vi "CRYDataView Main.vi"() -> ()   [LabVIEW 2013]
uses:
  <vilib>/Utility/miscctls.llb/LVRectTypeDef.ctl
  CRYView Global.vi
  CRYMainGlobal.vi
  CRYNew View Global.vi
  SubVI/CRYMain Sub Window Global.vi
panel:
  in  "pGraphMain VI Ref":refnum<vi>
  in  "Align":bool
  in  "bChangeState":bool
  in  "nIDFParent":i32
  in  "nSizeOver":i32
  in  "sAddGraphName":string="DataView"
  in  "Y2_Autoscale":bool
  in  "Y1_Autoscale":bool
  in  "X_Autoscale":bool
  in  "PreviewShowOnOff":bool
  in  "LegendShowOnOff":bool
  in  "Digital":bool
  in  "Intensity":bool
  in  "Octave":bool
  in  "Picture":bool
  in  "Polar":bool
  in  "Result":bool
  in  "Table":bool
  in  "Text":bool
  in  "Wave":bool
  in  "XY":bool
  in  "CursorShowOnOff":bool
  in  "sViewType":string="DataView"
  in  "sCloseMode":string="DataView"
  in  "AttachView":bool
  in  "sAddGraphLRAB":string="DataView"
  in  "Add Graph":bool
  in  "StateOut":bool
  in  "sTitle":string="DataView"
  in  "nIDV":i32
  in  "Revert":bool
  in  "Property":bool
  in  "TitleShowOnOff":bool
  in  "Save As":bool
  in  "Load":bool
  in  "stop":bool
  in  "cNewBootVIEW":T1
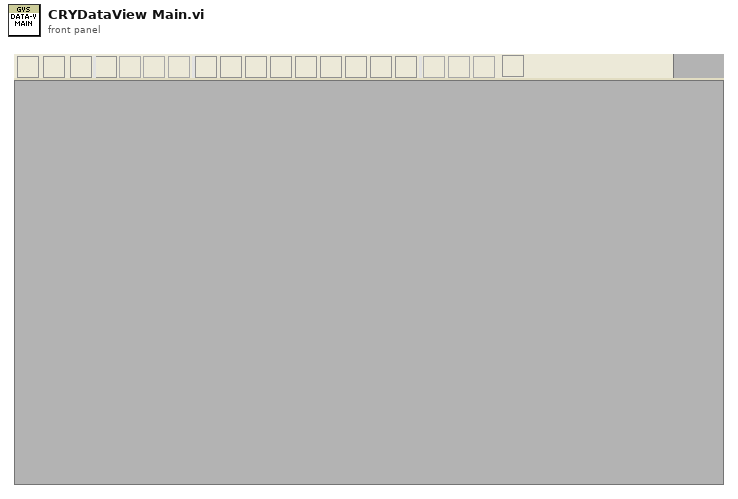
[diagram p1: front panel]
types:
  T1 = cluster{"sAction":string, "sType":string, "sQueueName":string, "sGraphName":string, "sData":string, "nData":i32, "pVIRef":refnum<vi>, "pSPRef":refnum<vi>}
  T2 = enum32{"English", "Chinese", "Korean", "Japanese", "Russian", "Chinese traditional"}
  T3 = typedef "LVRectTypeDef.ctl" = cluster{"Left":i16, "Top":i16, "Right":i16, "Bottom":i16}
  T4 = enum8{"Enabled", "Disabled", "Disabled and Grayed Out"}
  T5 = typedef "LVBoundsTypeDef.ctl" = cluster{"Width":u32, "Height":u32}
  T6 = cluster{"nID":i32, "sName":string, "sType":string, "sProperty":string, "sTemplet":string, "sDocking":string, "pVIRef":refnum<vi>, "pSPRef":refnum<vi>, "pRefTemplet":refnum<vi>, "pRefSplitter":refnum<vi>[], "nPosSplitter":i32[], "pRefSP":refnum<vi>[], "nSPID":i32[], "sSPDock":string[], "nIDFrame":i32[], "nIDPanel":i32[], "nActiveFrame":i32, "nCountFrame":i32, "cFrame":cluster{"nID":i32, "sName":string, "sType":string, "sTitle":string, "sIcon":string, "pVIRef":refnum<vi>, "pSPRef":refnum<vi>, "cWiin":cluster{"sName":string, "sType":string, "pVIRef":refnum<vi>, "sData":string}, "cTab":cluster{"sTitle":string, "sIcon":string, "pSpliter":refnum<vi>, "nAvtivePage":i32, "nIDPage":i32[], "nIDFrame":i32[]}, "sData":string}[], "sData":string, "sSplitterName":string[]}
  T7 = cluster{"nType":i32, "nParent":i32, "pVIW":refnum<vi>, "pSPW":refnum<vi>, "nTypeF":i32, "pVIF":refnum<vi>, "pSPF":refnum<vi>, "nIDSpliter":i32, "nProperty":i32, "Bound":T3, "nID":i32, "nData":i32, "sData":string, "pWVI":refnum<vi>, "sTitle":string, "cPages":cluster{"nPage":i32, "sTitle":string, "sIcon":string, "pVI":refnum<vi>, "nID":i32}[], "pTab":refnum<vi>, "nIDPages":i32[], "pSPT":refnum<vi>, "sTemp":string, "nDockID":i32, "nDockLR":i32, "sIcon":string}
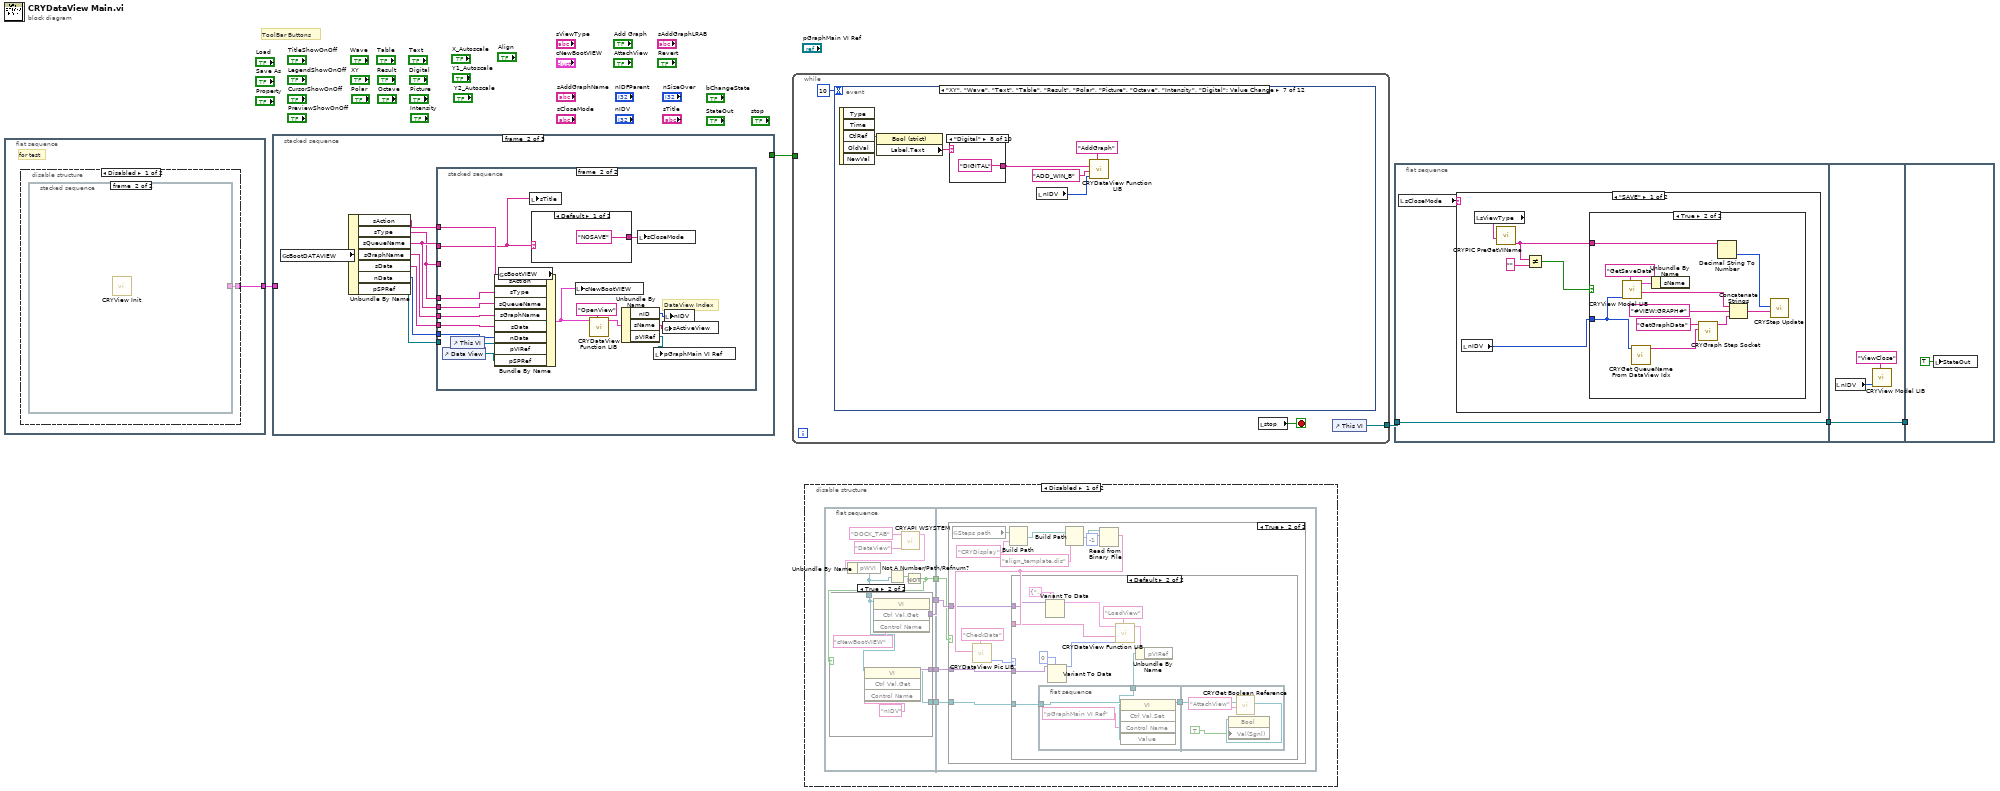
[diagram p0: block diagram]
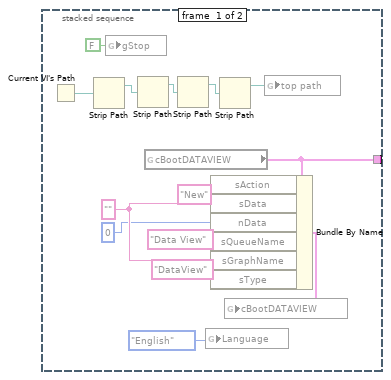
[diagram p6: hidden frame]
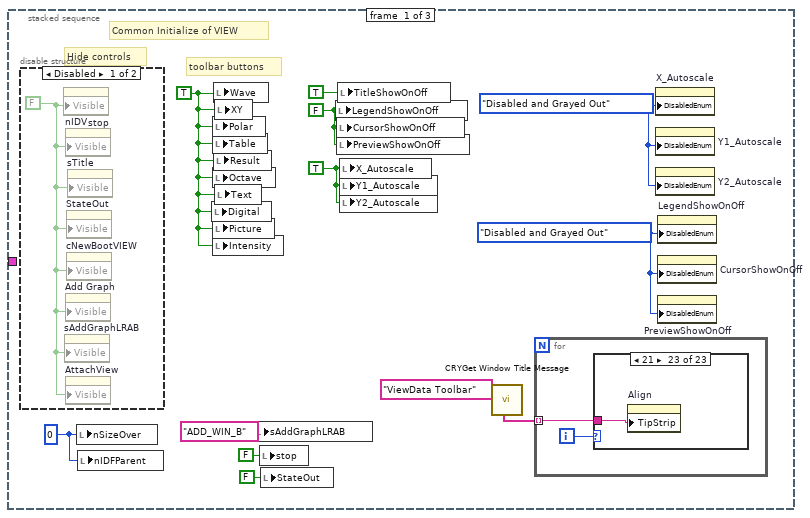
[diagram p10: hidden frame]
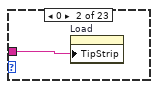
[diagram p13: hidden frame]
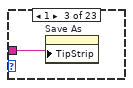
[diagram p14: hidden frame]
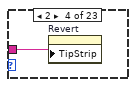
[diagram p15: hidden frame]
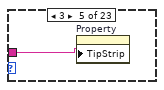
[diagram p16: hidden frame]
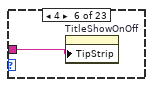
[diagram p17: hidden frame]
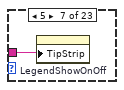
[diagram p18: hidden frame]
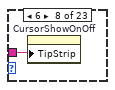
[diagram p19: hidden frame]
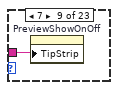
[diagram p20: hidden frame]
diagram:
  # "ToolBar Buttons"
  n1 = flat-sequence {
    tunnel: [w6] -> w1
    frame #0 {
      # "for test"
      n2 = disable-structure shown="Disabled" {
        disable-tunnel: [w7 _] -> w6
        frame Disabled {
          n3 = stacked-sequence {
            tunnel: [w8 _] -> w7
            frame #0 {
              w15 = "" ("sData")
              n4 = Current VI's Path() -> (path=w21:path)
              n5 = Strip Path(path=w21) -> (stripped path=w20:path)  [unwired: 1 out]
              n6 = global write "CRYMain Sub Window Global.vi" "gStop"(FALSE ("gStop")) -> ()
              n7 = Strip Path(path=w20) -> (stripped path=w19:path)  [unwired: 1 out]
              n8 = global read "CRYView Global.vi" "cBootDATAVIEW"() -> (w8:T1)
              n9 = Strip Path(path=w19) -> (stripped path=w18:path)  [unwired: 1 out]
              n10 = global write "CRYMainGlobal.vi" "Language"(T2."English" ("Language")) -> ()
              n11 = Bundle By Name(cluster=w8, "sAction"="New", "sData"=w15, "nData"=0, "sQueueName"="Data View", "sGraphName"=w15, "sType"="DataView") -> (w10:T1)
              n12 = Strip Path(path=w18) -> (stripped path=w17:path)  [unwired: 1 out]
              n13 = global write "CRYView Global.vi" "cBootDATAVIEW"(w10) -> ()
              n14 = global write "CRYMainGlobal.vi" "top path"(w17) -> ()
            }
            frame #1 {
              n15 = call "CRYView Init.vi"() -> ()  [unwired: 12 in]
            }
          }
        }
        frame Enabled {
        }
      }
    }
  }
  n16 = stacked-sequence {
    tunnel: [_ _ w97] -> w4
    tunnel: w1 -> [_ _ _]
    frame #0 {
      w23 = 0 ("nSizeOver")
      w24 = FALSE ("TitleShowOnOff")
      w25 = T4."Disabled and Grayed Out" ("Disabled")
      w26 = T4."Disabled and Grayed Out" ("Disabled")
      w27 = TRUE ("TitleShowOnOff")
      w29 = TRUE
      # "Hide controls"
      # "Common Initialize of VIEW"
      # "toolbar buttons"
      n17 = disable-structure shown="Disabled" {
        frame Disabled {
          w34 = FALSE
          n18 = property on="stop" class="Bool (strict)"("Visible"=w34) -> ()  [unwired: 2 in, 2 out]
          n19 = property on="sAddGraphLRAB" class="Str"("Visible"=w34) -> ()  [unwired: 2 in, 2 out]
          n20 = property on="nIDV" class="DigNum (strict)"("Visible"=w34) -> ()  [unwired: 2 in, 2 out]
          n21 = property on="Add Graph" class="Bool (strict)"("Visible"=w34) -> ()  [unwired: 2 in, 2 out]
          n22 = property on="AttachView" class="Bool (strict)"("Visible"=w34) -> ()  [unwired: 2 in, 2 out]
          n23 = property on="StateOut" class="Bool (strict)"("Visible"=w34) -> ()  [unwired: 2 in, 2 out]
          n24 = property on="cNewBootVIEW" class="Clust (strict)"("Visible"=w34) -> ()  [unwired: 2 in, 2 out]
          n25 = property on="sTitle" class="Str"("Visible"=w34) -> ()  [unwired: 2 in, 2 out]
        }
        frame Enabled {
        }
      }
      n26 = local write "nSizeOver"(w23) -> ()
      n27 = local write "nIDFParent"(w23) -> ()
      n28 = local write "Digital"(w29) -> ()
      n29 = local write "Polar"(w29) -> ()
      n30 = local write "Table"(w29) -> ()
      n31 = local write "Octave"(w29) -> ()
      n32 = local write "Picture"(w29) -> ()
      n33 = local write "Intensity"(w29) -> ()
      n34 = local write "Wave"(w29) -> ()
      n35 = local write "Result"(w29) -> ()
      n36 = local write "XY"(w29) -> ()
      n37 = local write "Text"(w29) -> ()
      n38 = local write "sAddGraphLRAB"("ADD_WIN_B" ("sAddGraphLRAB")) -> ()
      n39 = local write "stop"(FALSE ("stop")) -> ()
      n40 = local write "StateOut"(FALSE ("StateOut")) -> ()
      n41 = local write "LegendShowOnOff"(w24) -> ()
      n42 = local write "CursorShowOnOff"(w24) -> ()
      n43 = local write "PreviewShowOnOff"(w24) -> ()
      n44 = local write "TitleShowOnOff"(TRUE ("TitleShowOnOff")) -> ()
      n45 = local write "X_Autoscale"(w27) -> ()
      n46 = local write "Y1_Autoscale"(w27) -> ()
      n47 = local write "Y2_Autoscale"(w27) -> ()
      n48 = call "CRYGet Window Title Message.vi"("Kind"="ViewData Toolbar") -> ("Tip Strip"=w31:string[])  [unwired: 5 in, 5 out]
      n49 = for {
        tunnel: w31 -> [w35] mode=indexing
        i -> [w36]
        n50 = case shown="21" w36 {
          tunnel: w35 -> [_ w37 w38 w39 w40 w41 w42 w43 w44 w45 w46 w47 w48 w49 w50 w51 w52 w53 w54 w55 w56 w57 w58]
          frame Default {
          }
          frame 0 {
            n51 = property on="Load" class="Bool (strict)"("TipStrip"=w37) -> ()  [unwired: 2 in, 2 out]
          }
          frame 1 {
            n52 = property on="Save As" class="Bool (strict)"("TipStrip"=w38) -> ()  [unwired: 2 in, 2 out]
          }
          frame 2 {
            n53 = property on="Revert" class="Bool (strict)"("TipStrip"=w39) -> ()  [unwired: 2 in, 2 out]
          }
          frame 3 {
            n54 = property on="Property" class="Bool (strict)"("TipStrip"=w40) -> ()  [unwired: 2 in, 2 out]
          }
          frame 4 {
            n55 = property on="TitleShowOnOff" class="Bool (strict)"("TipStrip"=w41) -> ()  [unwired: 2 in, 2 out]
          }
          frame 5 {
            n56 = property on="LegendShowOnOff" class="Bool (strict)"("TipStrip"=w42) -> ()  [unwired: 2 in, 2 out]
          }
          frame 6 {
            n57 = property on="CursorShowOnOff" class="Bool (strict)"("TipStrip"=w43) -> ()  [unwired: 2 in, 2 out]
          }
          frame 7 {
            n58 = property on="PreviewShowOnOff" class="Bool (strict)"("TipStrip"=w44) -> ()  [unwired: 2 in, 2 out]
          }
          frame 8 {
            n59 = property on="Wave" class="Bool (strict)"("TipStrip"=w45) -> ()  [unwired: 2 in, 2 out]
          }
          frame 9 {
            n60 = property on="XY" class="Bool (strict)"("TipStrip"=w46) -> ()  [unwired: 2 in, 2 out]
          }
          frame 10 {
            n61 = property on="Polar" class="Bool (strict)"("TipStrip"=w47) -> ()  [unwired: 2 in, 2 out]
          }
          frame 11 {
            n62 = property on="Table" class="Bool (strict)"("TipStrip"=w48) -> ()  [unwired: 2 in, 2 out]
          }
          frame 12 {
            n63 = property on="Result" class="Bool (strict)"("TipStrip"=w49) -> ()  [unwired: 2 in, 2 out]
          }
          frame 13 {
            n64 = property on="Octave" class="Bool (strict)"("TipStrip"=w50) -> ()  [unwired: 2 in, 2 out]
          }
          frame 14 {
            n65 = property on="Text" class="Bool (strict)"("TipStrip"=w51) -> ()  [unwired: 2 in, 2 out]
          }
          frame 15 {
            n66 = property on="Digital" class="Bool (strict)"("TipStrip"=w52) -> ()  [unwired: 2 in, 2 out]
          }
          frame 16 {
            n67 = property on="Picture" class="Bool (strict)"("TipStrip"=w53) -> ()  [unwired: 2 in, 2 out]
          }
          frame 17 {
            n68 = property on="Intensity" class="Bool (strict)"("TipStrip"=w54) -> ()  [unwired: 2 in, 2 out]
          }
          frame 18 {
            n69 = property on="X_Autoscale" class="Bool (strict)"("TipStrip"=w55) -> ()  [unwired: 2 in, 2 out]
          }
          frame 19 {
            n70 = property on="Y1_Autoscale" class="Bool (strict)"("TipStrip"=w56) -> ()  [unwired: 2 in, 2 out]
          }
          frame 20 {
            n71 = property on="Y2_Autoscale" class="Bool (strict)"("TipStrip"=w57) -> ()  [unwired: 2 in, 2 out]
          }
          frame 21 {
            n72 = property on="Align" class="Bool (strict)"("TipStrip"=w58) -> ()  [unwired: 2 in, 2 out]
          }
        }
      }
      n73 = property on="X_Autoscale" class="Bool (strict)"("DisabledEnum"=w26) -> ()  [unwired: 2 in, 2 out]
      n74 = property on="Y1_Autoscale" class="Bool (strict)"("DisabledEnum"=w26) -> ()  [unwired: 2 in, 2 out]
      n75 = property on="Y2_Autoscale" class="Bool (strict)"("DisabledEnum"=w26) -> ()  [unwired: 2 in, 2 out]
      n76 = property on="LegendShowOnOff" class="Bool (strict)"("DisabledEnum"=w25) -> ()  [unwired: 2 in, 2 out]
      n77 = property on="CursorShowOnOff" class="Bool (strict)"("DisabledEnum"=w25) -> ()  [unwired: 2 in, 2 out]
      n78 = property on="PreviewShowOnOff" class="Bool (strict)"("DisabledEnum"=w25) -> ()  [unwired: 2 in, 2 out]
    }
    frame #1 {
      n79 = global read "CRYView Global.vi" "cBootDATAVIEW"() -> (w59:T1)
      n80 = Unbundle By Name(w59) -> ("sAction"=w62:string, "sType"=w61:string, "sQueueName"=w66:string, "sGraphName"=w65:string, "sData"=w64:string, "nData"=w63:i32, "pSPRef"=w60:refnum<vi>)
      n81 = stacked-sequence {
        tunnel: w62 -> [_ w86]
        tunnel: w66 -> [_ w79]
        tunnel: w63 -> [_ w90]
        tunnel: w64 -> [_ w91]
        tunnel: w65 -> [_ w92]
        tunnel: w66 -> [_ w93]
        tunnel: w61 -> [_ w94]
        tunnel: w61 -> [_ _]
        tunnel: w60 -> [w69 _]
        frame #0 {
          n82 = property class="SubPnl"(reference=w69) -> (error out=w68:errorcluster, "Bounds"=w67:T5)  [unwired: 1 in, 1 out]
          n83 = case shown="No Error" w68 {
            tunnel: w67 -> [w77 _]
            frame No Error {
              w72 = i16 0 ("Left")
              n84 = Unbundle By Name(w77) -> ("Width"=w74:u32, "Height"=w73:u32)
              n85 = Bundle By Name(cluster=T3 {"Left"=0, "Top"=0, "Right"=0, "Bottom"=0} ("Front Panel Window:Panel Bounds"), "Left"=w72, "Top"=w72, "Right"=w74, "Bottom"=w73) -> (w71:T3)
              n86 = control-ref of="This VI"() -> (w76:refnum<vi>)
              n87 = property class="VI"(reference=w76, "Front Panel.PanelBounds"=w71) -> (error out=w70:errorcluster)  [unwired: 1 in, 1 out]
              n88 = case shown="No Error" w70 {
                frame No Error {
                }
                frame Error {
                }
              }
            }
            frame Error {
            }
          }
        }
        frame #1 {
          # "DataView Index"
          n89 = control-ref of="Data View"() -> (w88:refnum<vi>)
          n90 = control-ref of="This VI"() -> (w84:refnum<vi>)
          n91 = global read "CRYView Global.vi" "cBootVIEW"() -> (w89:T1)
          n92 = Bundle By Name(cluster=w89, "sAction"=w86, "sType"=w94, "sQueueName"=w93, "sGraphName"=w92, "sData"=w91, "nData"=w90, "pVIRef"=w84, "pSPRef"=w88) -> (w87:T1)
          n93 = local write "sTitle"(w79) -> ()
          n94 = case shown="Default" w79 {
            tunnel: ["NOSAVE" "SAVE"] -> w85
            frame Default {
            }
            frame "ViewStep" {
            }
          }
          n95 = local write "cNewBootVIEW"(w87) -> ()
          n96 = call "CRYDataView Function LIB.vi"("sAction"="OpenView", "cBootVIEW"=w87) -> ("cView_Out"=w82:T6)  [unwired: 7 in, 2 out]
          n97 = Unbundle By Name(w82) -> ("nID"=w81:i32, "sName"=w80:string, "pVIRef"=w78:refnum<vi>)
          n98 = local write "sCloseMode"(w85) -> ()
          n99 = local write "pGraphMain VI Ref"(w78) -> ()
          n100 = global write "CRYView Global.vi" "sActiveView"(w80) -> ()
          n101 = local write "nIDV"(w81) -> ()
        }
      }
    }
    frame #2 {
      w97 = TRUE
      n102 = local write "StateOut"(w97) -> ()
    }
  }
  n103 = while {
    tunnel: [w99] -> w5
    tunnel: w4 -> [_]
    stop <- w98 stop-if-true
    n104 = event shown="[6] \"XY\", \"Wave\", \"Text\", \"Table\", \"Result\", \"Polar\", \"Picture\", \"Octave\", \"Intensity\", \"Digital\": Value Change" {
      selector: _ -> [_ _ _ _ _ _ _ _ _ _ _ _]
      dyn-events: _ -> [_ _ _ _ _ _ _ _ _ _ _ _]
      timeout: 10 -> [_ _ _ _ _ _ _ _ _ _ _ _]
      event Timeout {
        n105 = event-data() -> ()  [unwired: 1 in, 2 out]
      }
      event "Load": Value Change {
        n106 = event-data() -> ()  [unwired: 1 in, 5 out]
        n107 = global read "CRYMainGlobal.vi" "Steps path"() -> (w104:path)
        n108 = Build Path(base path=w104, name or relative path="CRYDisplay") -> (appended path=w103:path)
        n109 = call "CRYStep Read.vi"("Category Name"="Display" ("Step File Name"), "Step File Path"=w103) -> ("status"=w101:bool, "Flatten Step"=w102:string)  [unwired: 2 in, 4 out]
        n110 = case shown="True" w101 {
          tunnel: w102 -> [_ w107]
          frame False {
          }
          frame True {
            n111 = call "CRYDataView Pic LIB.vi"("sAction"="CheckData", "sOption"=w107) -> ("nData_Out"=w108:i32)  [unwired: 7 in, 2 out]
            n112 = case shown="Default" w108 {
              tunnel: w107 -> [_ w114]
              frame -1 {
              }
              frame Default {
                n113 = local read "nIDV"() -> (w112:i32)
                n114 = local read "cNewBootVIEW"() -> (w113:T1)
                n115 = call "CRYDataView Function LIB.vi"("sAction"="LoadView", "nData"=w112, "sData"=w114, "cBootVIEW"=w113) -> ("cView_Out"=w111:T6)  [unwired: 5 in, 2 out]
                n116 = Unbundle By Name(w111) -> ("pVIRef"=w110:refnum<vi>)
                n117 = flat-sequence {
                  tunnel: w110 -> [w116]
                  frame #0 {
                    n118 = local write "pGraphMain VI Ref"(w116) -> ()
                  }
                  frame #1 {
                    n119 = property on="AttachView" class="Bool (strict)"("Val(Sgnl)"=TRUE ("Value (Signaling)")) -> ()  [unwired: 2 in, 2 out]
                  }
                }
              }
            }
          }
        }
      }
      event "Save As": Value Change {
        n120 = event-data() -> ()  [unwired: 1 in, 5 out]
        n121 = local read "sViewType"() -> (w118:string)
        n122 = local read "nIDV"() -> (w119:i32)
        n123 = call "CRYDataView Function LIB.vi"("sAction"="SaveView", "nData"=w119, "sOption"=w118) -> ()  [unwired: 6 in, 3 out]
      }
      event "Revert": Value Change {
        n124 = event-data() -> ()  [unwired: 1 in, 5 out]
        n125 = local read "cNewBootVIEW"() -> (w121:T1)
        n126 = local read "nIDV"() -> (w122:i32)
        n127 = call "CRYDataView Function LIB.vi"("sAction"="ReloadView", "nData"=w122, "cBootVIEW"=w121) -> ()  [unwired: 6 in, 3 out]
      }
      event "TitleShowOnOff": Value Change {
        n128 = event-data() -> ()  [unwired: 1 in, 5 out]
        n129 = local read "nIDV"() -> (w124:i32)
        n130 = call "CRYDataView Function LIB.vi"("sAction"="TitleBarOnOff", "nData"=w124) -> ()  [unwired: 7 in, 3 out]
      }
      event "CursorShowOnOff", "LegendShowOnOff", "PreviewShowOnOff", "Property": Value Change {
        n131 = event-data() -> ("CtlRef"=w137:refnum<vi>, "OldVal"=w129:bool)  [unwired: 1 in, 3 out]
        n132 = property class="Bool (strict)"(reference=w137) -> ("Label.Text"=w136:string)  [unwired: 1 in, 2 out]
        n133 = local read "nIDV"() -> (w126:i32)
        n134 = case shown="\"CursorShowOnOff\"" w136 {
          tunnel: ["LEGEND_VIEW" ("input 1") "CURSOR_VIEW" ("input 1") "PREVIEW_VIEW" ("input 1") "DA_PROPERTY" ("input 1")] -> w132
          frame "LegendShowOnOff", Default {
          }
          frame "CursorShowOnOff" {
          }
          frame "PreviewShowOnOff" {
          }
          frame "Property" {
          }
        }
        n135 = Select(t=1, s=w129, f=-1) -> (s? t:f=w128:i32)
        n136 = call "CRYGet QueueName From DataView Idx.vi"("DataView Idx"=w126) -> ("DataView sQueueName"=w127:string)  [unwired: 10 in]
        n137 = Obtain Queue(name (unnamed)=w127, element data type="" ("Action Type")) -> (queue out=w133:refnum<queue>)  [unwired: 3 in, 2 out]
        n138 = Format Into String(w132, w132, w128, w126) -> (resulting string=w134:string)  [unwired: 3 in, 1 out]
        n139 = Enqueue Element(queue=w133, element=w134) -> ()  [unwired: 1 in, 4 out]
      }
      event "XY", "Wave", "Text", "Table", "Result", "Polar", "Picture", "Octave", "Intensity", "Digital": Value Change {
        n140 = event-data() -> ("CtlRef"=w142:refnum<vi>)  [unwired: 1 in, 4 out]
        n141 = property class="Bool (strict)"(reference=w142) -> ("Label.Text"=w143:string)  [unwired: 1 in, 2 out]
        n142 = case shown="\"Digital\"" w143 {
          tunnel: ["WAVE" "XY" "POLAR" "TABLE" "RESULT" "OCTAVE" "TEXT" "DIGITAL" "PICTURE" "INTENSITY"] -> w144
          frame "Wave", Default {
          }
          frame "XY" {
          }
          frame "Polar" {
          }
          frame "Table" {
          }
          frame "Result" {
          }
          frame "Octave" {
          }
          frame "Text" {
          }
          frame "Digital" {
          }
          frame "Picture" {
          }
          frame "Intensity" {
          }
        }
        n143 = local read "nIDV"() -> (w147:i32)
        n144 = call "CRYDataView Function LIB.vi"("sAction"="AddGraph", "nData"=w147, "sData"="ADD_WIN_B", "sOption"=w144) -> ()  [unwired: 5 in, 3 out]
      }
      event "X_Autoscale", "Y1_Autoscale", "Y2_Autoscale": Value Change {
        n145 = event-data() -> ("CtlRef"=w161:refnum<vi>)  [unwired: 1 in, 4 out]
        n146 = property class="Bool (strict)"(reference=w161) -> ("Label.Text"=w167:string)  [unwired: 1 in, 2 out]
        n147 = local read "nIDV"() -> (w159:i32)
        n148 = property class="Bool (strict)"(reference=w161) -> ("Value"=w162:bool)  [unwired: 1 in, 2 out]
        n149 = case shown="\"X_Autoscale\", Default" w167 {
          tunnel: ["X_AUTOSCALE" ("input 1") "Y1_AUTOSCALE" ("input 1") "Y2_AUTOSCALE" ("input 1")] -> w163
          frame "X_Autoscale", Default {
          }
          frame "Y1_Autoscale" {
          }
          frame "Y2_Autoscale" {
          }
        }
        n150 = Not(x=w162) -> (.not. x?=w160:bool)
        n151 = call "CRYGet QueueName From DataView Idx.vi"("DataView Idx"=w159) -> ("DataView sQueueName"=w158:string)  [unwired: 10 in]
        n152 = Select(t=1, s=w160, f=-1) -> (s? t:f=w164:i32)
        n153 = flat-sequence {
          tunnel: w163 -> [w171]
          tunnel: w158 -> [w170]
          tunnel: w164 -> [w169]
          tunnel: w159 -> [w168]
          frame #0 {
            n154 = Obtain Queue(name (unnamed)=w170, element data type="" ("Action Type")) -> (queue out=w172:refnum<queue>)  [unwired: 3 in, 2 out]
            n155 = Format Into String(w171, w171, w169, w168) -> (resulting string=w173:string)  [unwired: 3 in, 1 out]
            n156 = Enqueue Element(queue=w172, element=w173) -> ()  [unwired: 1 in, 4 out]
          }
        }
      }
      event "Align": Value Change {
        n157 = event-data() -> ()  [unwired: 1 in, 5 out]
        n158 = flat-sequence {
          frame #0 {
            n159 = global write "CRYNew View Global.vi" "g_WaitFlag"(TRUE ("g_WaitFlag")) -> ()
          }
          frame #1 {
            w180 = "VIEW_DATA_VIEW_TEMPLATE" ("input 1")
            w181 = 0 ("input 3")
            n160 = Obtain Queue(name (unnamed)="CRYMAIN_ACTION" ("YAxisTitle"), element data type="" ("Action Type")) -> (queue out=w179:refnum<queue>)  [unwired: 3 in, 2 out]
            n161 = Format Into String(w180, w180, w181, w181) -> (resulting string=w182:string)  [unwired: 3 in, 1 out]
            n162 = Enqueue Element(queue=w179, element=w182) -> ()  [unwired: 1 in, 4 out]
          }
        }
      }
      event "AttachView": Value Change {
        # "Fit problem"
        n163 = event-data() -> ()  [unwired: 1 in, 5 out]
        n164 = local read "pGraphMain VI Ref"() -> (w185:refnum<vi>)
        n165 = control-ref of="Data View"() -> (w186:refnum<vi>)
        n166 = invoke class="SubPnl" method="Insert VI"(reference=w186, "VI Ref"=w185) -> (reference out=w188:refnum<vi>, error out=w187:errorcluster)  [unwired: 2 in, 2 out]
        n167 = invoke class="SubPnl" method="FitControlToPane"(reference=w188, error in=w187) -> ()  [unwired: 1 in, 3 out]
      }
      event "bChangeState": Value Change {
        n168 = event-data() -> ("NewVal"=w193:bool)  [unwired: 1 in, 4 out]
        n169 = case shown="False" w193 {
          tunnel: [T4."Enabled" ("Disabled") T4."Disabled and Grayed Out" ("Disabled")] -> w192
          frame False {
          }
          frame True {
          }
        }
        n170 = control-ref of="Load"() -> (w191:refnum<vi>)
        n171 = control-ref of="Save As"() -> (w190:refnum<vi>)
        n172 = control-ref of="Property"() -> (w189:refnum<vi>)
        n173 = Build Array(w191, w190, w189) -> (w194:refnum<vi>[])
        n174 = for {
          tunnel: w194 -> [w196] mode=indexing
          tunnel: w192 -> [w195]
          n175 = property class="Bool (strict)"(reference=w196, "DisabledEnum"=w195) -> ()  [unwired: 1 in, 2 out]
        }
      }
      event Pane Size {
        w201 = 24
        n176 = event-data() -> ()  [unwired: 1 in, 5 out]
        n177 = local read "nSizeOver"() -> (w199:i32)
        n178 = control-ref of="Splitter"() -> (w200:refnum<vi>)
        n179 = property class="Splitter"(reference=w200) -> (reference out=w202:refnum<vi>, "Position"=w204:i32)  [unwired: 1 in, 1 out]
        n180 = Less?(x=w204, y=w201) -> (x < y?=w203:bool)
        n181 = case shown="True" w203 {
          tunnel: w202 -> [_ w249]
          tunnel: w201 -> [_ w251]
          tunnel: w199 -> [w205 _]
          frame False {
            n182 = disable-structure shown="Disabled" {
              disable-tunnel: w205 -> [w206 _]
              frame Disabled {
                n183 = case shown="Default" w206 {
                  frame 0 {
                  }
                  frame Default {
                    n184 = stacked-sequence {
                      seq-local: [w213 _ _] -> [_ w225 w235]
                      frame #0 {
                        n185 = local read "nIDV"() -> (w207:i32)
                        n186 = local read "nIDV"() -> (w214:i32)
                        n187 = call "CRYGet Active Graph Ref to DVIndex.vi"("DV Array index"=w207) -> ()  [unwired: 5 in, 6 out]
                        n188 = call "CRYDataView Function LIB.vi"("sAction"="GetViewByID", "nData"=w214) -> ("cView_Out"=w213:T6)  [unwired: 7 in, 2 out]
                        n189 = control-ref of="Data View"() -> (w210:refnum<vi>)
                        n190 = Unbundle By Name(w213) -> ("pSPRef"=w209:refnum<vi>)
                        n191 = invoke class="SubPnl" method="Remove VI"(reference=w209) -> (reference out=w212:refnum<vi>)  [unwired: 2 in, 2 out]
                        n192 = invoke class="SubPnl" method="FitControlToPane"(reference=w212) -> (error out=w208:errorcluster)  [unwired: 2 in, 2 out]
                        n193 = invoke class="SubPnl" method="Remove VI"(reference=w210, error in=w208) -> (reference out=w211:refnum<vi>)  [unwired: 1 in, 2 out]
                        n194 = invoke class="SubPnl" method="FitControlToPane"(reference=w211) -> ()  [unwired: 2 in, 3 out]
                      }
                      frame #1 {
                        n195 = control-ref of="Data View"() -> (w221:refnum<vi>)
                        n196 = Unbundle By Name(w225) -> ("pSPRef"=w218:refnum<vi>, "pRefTemplet"=w217:refnum<vi>, "pVIRef"=w224:refnum<vi>)
                        n197 = invoke class="SubPnl" method="Insert VI"(reference=w221, "VI Ref"=w224) -> (reference out=w223:refnum<vi>, error out=w222:errorcluster)  [unwired: 2 in, 2 out]
                        n198 = invoke class="SubPnl" method="FitControlToPane"(reference=w223, error in=w222) -> (error out=w216:errorcluster)  [unwired: 1 in, 2 out]
                        n199 = invoke class="SubPnl" method="Insert VI"(reference=w218, error in=w216, "VI Ref"=w217) -> (reference out=w219:refnum<vi>, error out=w220:errorcluster)  [unwired: 1 in, 2 out]
                        n200 = invoke class="SubPnl" method="FitControlToPane"(reference=w219, error in=w220) -> ()  [unwired: 1 in, 3 out]
                      }
                      frame #2 {
                        n201 = control-ref of="This VI"() -> (w236:refnum<vi>)
                        n202 = Unbundle By Name(w235) -> ("pRefTemplet"=w231:refnum<vi>)
                        n203 = property class="VI"(reference=w236) -> ("Front Panel.PanelBounds"=w239:T3)  [unwired: 1 in, 2 out]
                        n204 = property class="VI"(reference=w231) -> ("Front Panel.PanelBounds"=w232:T3)  [unwired: 1 in, 2 out]
                        n205 = Unbundle By Name(w232) -> ("Bottom"=w233:i16, "Top"=w234:i16)
                        n206 = Unbundle By Name(w239) -> ("Bottom"=w238:i16, "Top"=w237:i16)
                        n207 = Subtract(x=w233, y=w234) -> (x-y=w228:i16)
                        n208 = Subtract(x=w238, y=w237) -> (x-y=w230:i16)
                        n209 = Subtract(x=w230, y=24) -> (x-y=w227:i32)
                        n210 = Greater?(x=w228, y=w227) -> (0:w226:bool)
                        n211 = case shown="False" w226 {
                          frame False {
                            n212 = local write "nSizeOver"(0 ("nSizeOver")) -> ()
                          }
                          frame True {
                          }
                        }
                      }
                    }
                  }
                }
              }
              frame Enabled {
              }
            }
          }
          frame True {
            n213 = disable-structure shown="Disabled" {
              disable-tunnel: [w254 _] -> _
              disable-tunnel: _ -> [w253 _]
              disable-tunnel: [w252 _] -> w245
              frame Disabled {
                n214 = control-ref of="Data View"() -> (w255:refnum<vi>)
                n215 = invoke class="SubPnl" method="Remove VI"(reference=w255) -> (reference out=w252:refnum<vi>, error out=w254:errorcluster)  [unwired: 2 in, 1 out]
                n216 = case shown="No Error" w253 {
                  frame No Error {
                  }
                  frame Error {
                  }
                }
              }
              frame Enabled {
              }
            }
            n217 = property class="Splitter"(reference=w249, "Locked"=FALSE ("Splitter Position Locked")) -> (reference out=w248:refnum<vi>, error out=w242:errorcluster)  [unwired: 1 in]
            n218 = property class="Splitter"(reference=w248, error in=w242, "Position"=w251) -> (reference out=w246:refnum<vi>, error out=w241:errorcluster)
            n219 = property class="Splitter"(reference=w246, error in=w241, "Locked"=TRUE ("Splitter Position Locked")) -> (error out=w244:errorcluster)  [unwired: 1 out]
            n220 = disable-structure shown="Disabled" {
              disable-tunnel: w245 -> [w259 _]
              disable-tunnel: w244 -> [w258 w262]
              frame Disabled {
                n221 = local read "nIDV"() -> (w257:i32)
                n222 = call "CRYGet Active Graph Ref to DVIndex.vi"("DV Array index"=w257) -> ("Graph Main VIRef"=w256:refnum<vi>)  [unwired: 5 in, 5 out]
                n223 = invoke class="SubPnl" method="Insert VI"(reference=w259, error in=w258, "VI Ref"=w256) -> (reference out=w260:refnum<vi>)  [unwired: 1 in, 3 out]
                n224 = invoke class="SubPnl" method="FitControlToPane"(reference=w260) -> ()  [unwired: 2 in, 3 out]
              }
              frame Enabled {
                n225 = control-ref of="Data View"() -> (w263:refnum<vi>)
                n226 = invoke class="SubPnl" method="FitControlToPane"(reference=w263, error in=w262) -> (error out=w261:errorcluster)  [unwired: 1 in, 2 out]
                n227 = case shown="No Error" w261 {
                  frame No Error {
                  }
                  frame Error {
                  }
                }
              }
            }
            n228 = local write "nSizeOver"(1 ("nSizeOver")) -> ()
          }
        }
      }
    }
    n229 = local read "stop"() -> (w98:bool)
    n230 = control-ref of="This VI"() -> (w99:refnum<vi>)
  }
  n231 = disable-structure shown="Disabled" {
    frame Disabled {
      n232 = flat-sequence {
        tunnel: [w273] -> w267
        tunnel: [w272] -> w266
        tunnel: [w271] -> w265
        tunnel: [w268] -> w264
        tunnel: w267 -> [w286]
        tunnel: w266 -> [w285]
        tunnel: w265 -> [w284]
        tunnel: w264 -> [w283]
        frame #0 {
          n233 = call "CRYAPI WSYSTEM.vi"("sData"="DataView" ("Window Type"), "sAction"="DOCK_TAB") -> ("tFrame_Out"=w274:T7)  [unwired: 6 in, 3 out]
          n234 = Unbundle By Name(w274) -> ("pWVI"=w270:refnum<vi>)
          n235 = Not A Number/Path/Refnum?(number/path/refnum=w270) -> (NaN/Path/Refnum?=w269:bool)
          n236 = Not(x=w269) -> (.not. x?=w268:bool)
          n237 = case shown="True" w268 {
            tunnel: [_ w282] -> w273
            tunnel: [_ w281] -> w272
            tunnel: [_ w280] -> w271
            tunnel: w270 -> [_ w277]
            frame False {
            }
            frame True {
              n238 = invoke class="VI" method="Ctrl Val.Get"(reference=w277, "Control Name"="nIDV") -> (reference out=w280:refnum<vi>, "Get Control Value Variant"=w281:variant)  [unwired: 2 in, 2 out]
              n239 = invoke class="VI" method="Ctrl Val.Get"(reference=w277, "Control Name"="cNewBootVIEW") -> ("Get Control Value Variant"=w282:variant)  [unwired: 2 in, 3 out]
            }
          }
        }
        frame #1 {
          n240 = case shown="True" w283 {
            tunnel: w286 -> [_ w289]
            tunnel: w285 -> [_ w288]
            tunnel: w284 -> [_ w287]
            frame False {
            }
            frame True {
              n241 = global read "CRYMainGlobal.vi" "Steps path"() -> (w295:path)
              n242 = Build Path(base path=w295, name or relative path="CRYDisplay") -> (appended path=w294:path)
              n243 = Build Path(base path=w294, name or relative path="align_template.dis") -> (appended path=w292:path)
              n244 = Read from Binary File(10:-1 ("count (1)"), 11:w292) -> (2:w290:string)  [unwired: 4 in, 3 out]
              n245 = call "CRYDataView Pic LIB.vi"("sAction"="CheckData", "sOption"=w290) -> ("nData_Out"=w297:i32)  [unwired: 7 in, 2 out]
              n246 = case shown="Default" w297 {
                tunnel: w290 -> [_ w309]
                tunnel: w289 -> [_ w306]
                tunnel: w288 -> [_ w303]
                tunnel: w287 -> [_ w300]
                frame -1 {
                }
                frame Default {
                  n247 = flat-sequence {
                    tunnel: w307 -> [w313]
                    tunnel: w300 -> [w314]
                    tunnel: [w311] -> w299
                    tunnel: w299 -> [w318]
                    frame #0 {
                      n248 = invoke class="VI" method="Ctrl Val.Set"(reference=w314, "Control Name"="pGraphMain VI Ref", "Value"=w313) -> (reference out=w311:refnum<vi>)  [unwired: 2 in, 4 out]
                    }
                    frame #1 {
                      n249 = call "CRYGet Boolean Reference.vi"("Label Name"="AttachView", "VI Refnum"=w318) -> ("Boolean Ref"=w316:refnum<vi>)  [unwired: 7 in, 2 out]
                      n250 = property class="Bool"(reference=w316, "Val(Sgnl)"=TRUE ("Value (Signaling)")) -> ()  [unwired: 1 in, 2 out]
                    }
                  }
                  n251 = Variant To Data(type=T1 {"sAction"="", "sType"="", "sQueueName"="", "sGraphName"="", "sData"="", "nData"=0, "pVIRef"=refnum, "pSPRef"=refnum} ("cNewBootVIEW"), Variant=w306) -> (data=w304:T1)  [unwired: 1 in, 1 out]
                  n252 = Variant To Data(type=0, Variant=w303) -> (data=w301:i32)  [unwired: 1 in, 1 out]
                  n253 = call "CRYDataView Function LIB.vi"("sAction"="LoadView", "nData"=w301, "sData"=w309, "cBootVIEW"=w304) -> ("cView_Out"=w308:T6)  [unwired: 5 in, 2 out]
                  n254 = Unbundle By Name(w308) -> ("pVIRef"=w307:refnum<vi>)
                }
              }
            }
          }
        }
      }
    }
    frame Enabled {
    }
  }
  n255 = flat-sequence {
    tunnel: [w320] -> w2
    tunnel: w5 -> [w320]
    tunnel: [w339] -> w3
    tunnel: w2 -> [w339]
    tunnel: w3 -> [_]
    frame #0 {
      n256 = local read "sCloseMode"() -> (w319:string)
      n257 = case shown="\"SAVE\"" w319 {
        frame "SAVE" {
          n258 = local read "nIDV"() -> (w324:i32)
          n259 = local read "sViewType"() -> (w325:string)
          n260 = call "CRYPIC PreGetVIName.vi"("sVIName"=w325) -> ("sData_Out"=w323:string)  [unwired: 9 in, 1 out]
          n261 = Not Equal?(x=w323, y="") -> (x != y?=w321:bool)
          n262 = case shown="True" w321 {
            tunnel: w324 -> [_ w327]
            tunnel: w323 -> [_ w328]
            frame False {
            }
            frame True {
              n263 = call "CRYView Model LIB.vi"("sAction"="GetSaveData", "nData"=w327) -> ("sData_Out"=w330:string, "cView_Out"=w334:T6)  [unwired: 7 in, 1 out]
              n264 = call "CRYGet QueueName From DataView Idx.vi"("DataView Idx"=w327) -> ("DataView sQueueName"=w326:string)  [unwired: 10 in]
              n265 = Unbundle By Name(w334) -> ()  [unwired: 1 out]
              n266 = call "CRYGraph Step Socket.vi"("Queue Name"=w326, "sAction"="GetGraphData") -> ("sDataOut"=w331:string)  [unwired: 9 in]
              n267 = Decimal String To Number(string=w328) -> (number=w329:i32)  [unwired: 2 in, 1 out]
              n268 = Concatenate Strings(w330, "#VIEW:GRAPH#" ("regular expression"), w331) -> (w332:string)
              n269 = call "CRYStep Update.vi"("Seq-step setup"=w332, "Proper VI No"=w329) -> ()  [unwired: 5 in, 5 out]
            }
          }
        }
        frame Default {
        }
      }
    }
    frame #1 {
      n270 = local read "nIDV"() -> (w338:i32)
      n271 = call "CRYView Model LIB.vi"("sAction"="ViewClose", "nData"=w338) -> ()  [unwired: 7 in, 3 out]
    }
    frame #2 {
      n272 = local write "StateOut"(TRUE ("StateOut")) -> ()
    }
  }
